vi "Min-Max Limit Switch.vi"(9 "Lower Limit":bool, 10 "Upper Limit":bool, 11 "Input":dbl) -> (3 "Output":dbl)   [LabVIEW 2014]
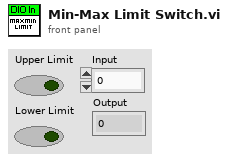
[diagram p1: front panel]
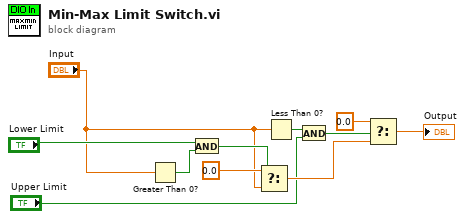
[diagram p0: block diagram]
diagram:
  n1 = Greater Than 0?(x="Input") -> (x > 0?=w11:bool)
  n2 = And(x="Lower Limit", y=w11) -> (x .and. y?=w9:bool)
  n3 = Select(t=0.0, s=w9, f="Input") -> (s? t:f=w5:dbl)
  n4 = Less Than 0?(x="Input") -> (x < 0?=w10:bool)
  n5 = And(x=w10, y="Upper Limit") -> (x .and. y?=w6:bool)
  n6 = Select(t=0.0, s=w6, f=w5) -> (s? t:f=→"Output":dbl)
